vi "Add Elements to Enum.vi"(10 "Item to Add":string[](array[string]), 11 "Typedef Enum Control Filepath (.ctl)":path) -> ()   [LabVIEW 2019]
doc: "This VI will show you how to programmatically add elements to an enum or a ring.\nYou cannot run this code if the actual control is in memory. This means that you cannot change the control and use it at the same time."
panel:
  # "Overview: This VI will show you how to programmatically add elements to an enum or a ring.\nRequirements: LabVIEW 2012 (or compatible)\nInstructions:\n1. Open the enum or  ring control (.ctl) you want to add elements to (i.e. Enum Control.ctl) \n2. Specify the filepath of the control opened\n3. Run this VI and see the new elements in the opened control."
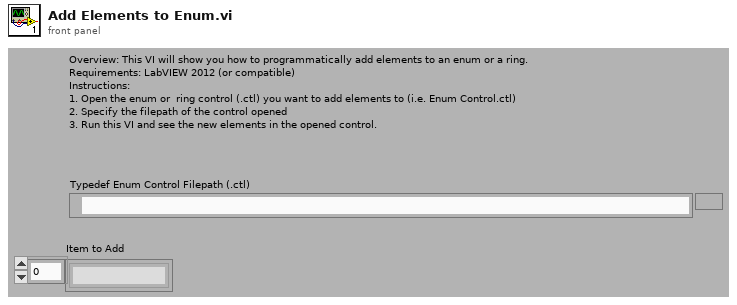
[diagram p1: front panel]
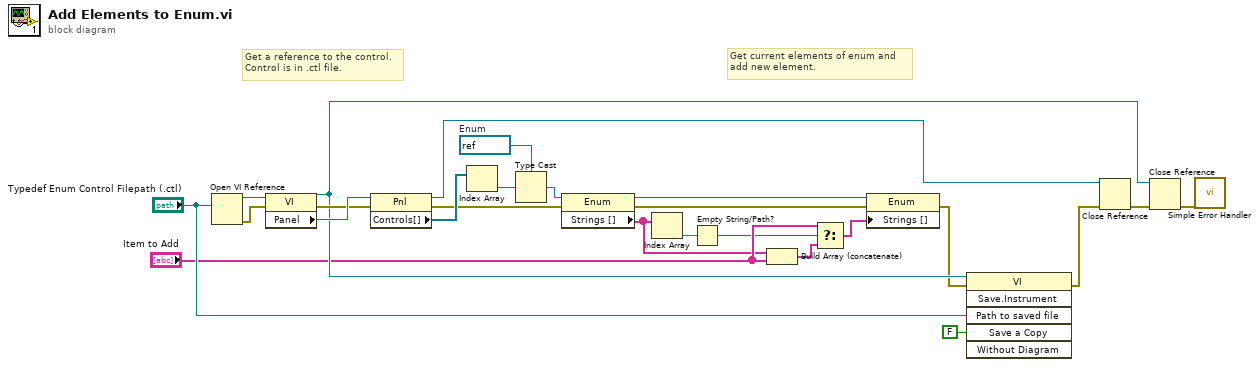
[diagram p0: block diagram]
diagram:
  w23 = refnum<vi> refnum  # Enum
  # "Get current elements of enum and\nadd new element."
  # "Get a reference to the control.\nControl is in .ctl file."
  n1 = Open VI Reference(vi path="Typedef Enum Control Filepath (.ctl)") -> (vi reference=w12:refnum<vi>, error out=w15:errorcluster)  [unwired: 5 in]
  n2 = property class="VI"(reference=w12, error in=w15) -> (reference out=w11:refnum<vi>, error out=w22:errorcluster, "Panel"=w25:refnum<vi>)
  n3 = property class="Pnl"(reference=w25, error in=w22) -> (reference out=w14:refnum<vi>, error out=w21:errorcluster, "Controls[]"=w24:refnum<vi>[])
  n4 = Index Array(array=w24) -> (element=w13:refnum<vi>)  [unwired: 1 in]
  n5 = Type Cast(type=w23, x=w13) -> (*(type *) &x=w16:refnum<vi>)
  n6 = property class="Enum"(reference=w16, error in=w21) -> (reference out=w19:refnum<vi>, error out=w18:errorcluster, "Strings []"=w1:string[])
  n7 = Index Array(array=w1) -> (element=w3:string)  [unwired: 1 in]
  n8 = Empty String/Path?(string/path=w3) -> (empty?=w2:bool)
  n9 = Build Array (concatenate)(w1, "Item to Add") -> (w5:string[])
  n10 = Select(t="Item to Add", s=w2, f=w5) -> (s? t:f=w4:string[])
  n11 = property class="Enum"(reference=w19, error in=w18, "Strings []"=w4) -> (error out=w10:errorcluster)  [unwired: 1 out]
  n12 = invoke class="VI" method="Save.Instrument"(reference=w11, error in=w10, "Path to saved file"="Typedef Enum Control Filepath (.ctl)", "Save a Copy"=FALSE) -> (error out=w9:errorcluster)  [unwired: 2 in, 5 out]
  n13 = Close Reference(reference=w14, error in (no error)=w9) -> (error out=w20:errorcluster)
  n14 = Close Reference(reference=w11, error in (no error)=w20) -> (error out=w17:errorcluster)
  n15 = call <vilib>:"Simple Error Handler.vi"("error in (no error)"=w17) -> ()  [unwired: 4 in, 5 out]
